vi "Begin.vi"   [LabVIEW 2011]
doc: "Called before other user functions, this VI is expected to open initial I/O refnums, load in file data, and do all program initialization. Notice that the <B>error out</B> terminal is simply used for data flow. Wiring it to other structures or subVIs ensures that this VI runs first."
uses:
  <vilib>/Rock Robotics/SystemInterfaces/DIO/FPGA_DIOPWMChannel.ctl
  <vilib>/Rock Robotics/SystemInterfaces/AI/FPGA_AIChannel.ctl
  <vilib>/Rock Robotics/WPI/Joystick/WPI_JoystickDeviceEnum.ctl
  Global.vi
  <vilib>/Rock Robotics/WPI/RobotDrive/WPI_RobotDriveOpen4MotorWithJaguar.vi
  Pivot Drive.lvlib
types:
  T1 = typedef "WPI_JoystickDeviceEnum.ctl" = enum16{"USB 1", "USB 2", "USB 3", "USB 4", "Kinect 1", "Kinect 2"}
  T2 = typedef "FPGA_AIChannel.ctl" = enum8{"AI 1", "AI 2", "AI 3", "AI 4", "AI 5", "AI 6", "AI 7", "AI 8", "Invalid"}
  T3 = typedef "FPGA_DIOPWMChannel.ctl" = enum8{"PWM 1", "PWM 2", "PWM 3", "PWM 4", "PWM 5", "PWM 6", "PWM 7", "PWM 8", "PWM 9", "PWM 10", "Invalid"}
  T4 = typedef "WPI_RobotDriveDevRef.ctl" = cluster{"DevStatus":errorcluster, "Motors[]":T5[], "Square Inputs":bool, "Max Output":dbl, "Isochronous":bool}
  T5 = typedef "WPI_MotorControlDeviceRef.ctl" = cluster{"DeviceStatus":errorcluster, "Type":enum16{"PWM", "CAN"}, "PWM":cluster{"Digital Module":T6, "PWM Channel":T3, "DeadBand":T7}, "CAN":cluster{"Device Number":u8, "Control Mode":T8, "Semaphore":T9, "Max Vout":dbl}, "Invert":bool, "TransformRef":T10, "InvTransformRef":T10}
  T6 = typedef "FPGA_TypedefDigitalModule.ctl" = enum16{"Digital Module 1", "Digital Module 2"}
  T7 = typedef "WPI_PWMDeadband.ctl" = cluster{"Name":string, "maxPositivePwm":i32, "minPositivePwm":i32, "centerPwm":i32, "maxNegativePwm":i32, "minNegativePwm":i32, "angularRange":u16}
  T8 = typedef "WPI_CANJaguar_ControlMode.ctl" = enum8{"Percent VBus", "Current", "Speed", "Position", "Voltage"}
  T9 = typedef "Semaphore RefNum" = refnum<k1>
  T10 = typedef "WPI_PWMTransform_ConPane.ctl" = refnum<vi>
  T11 = typedef "WPI_AnalogChannelDevRef.ctl" = cluster{"DevStatus":errorcluster, "Analog Module":T12, "Analog Channel":T2}
  T12 = typedef "FPGA_TypedefAnalogModule.ctl" = enum16{"Analog Module 1", "Analog Module 2"}
  T13 = typedef "WPI_JoystickDevRef.ctl" = cluster{"Device":T1}
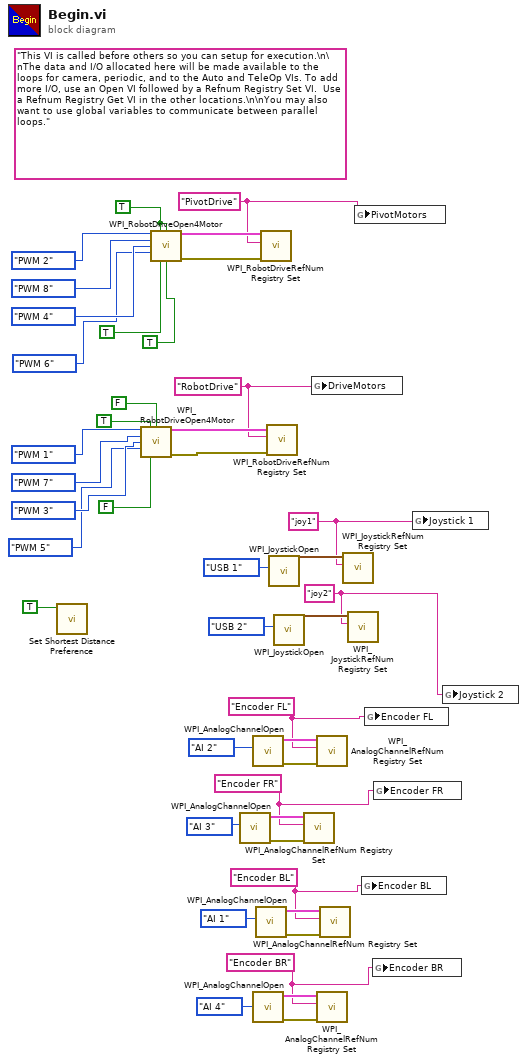
[diagram p0: block diagram]
diagram:
  w2 = TRUE ("Rear Left Motor Inverted")
  w24 = "joy2"
  w25 = "joy1"
  w16 = "Encoder BR" ("refnum name")
  w17 = "Encoder BL" ("refnum name")
  w18 = "Encoder FR" ("refnum name")
  w19 = "Encoder FL" ("refnum name")
  w20 = "RobotDrive" ("refnum name")
  w21 = "PivotDrive" ("refnum name")
  (unwired) "This VI is called before others so you can setup for execution.\n\nThe data and I/O allocated here will be made available to the loops for camera, periodic, and to the Auto and TeleOp VIs. To add more I/O, use an Open VI followed by a Refnum Registry Set VI.  Use a Refnum Registry Get VI in the other locations.\n\nYou may also want to use global variables to communicate between parallel loops."
  n1 = call "Set Shortest Distance Preference.vi"("Use Shortest Distance Relative?"=TRUE) -> ()  [unwired: 11 out]
  n2 = call-poly <vilib>:"WPI_RobotDriveOpen4Motor.vi"("Rear Left Motor"=FPGA_DIOPWMChannel."PWM 1", "Rear Left Motor Inverted"=TRUE ("Front Left Motor Inverted"), "Rear Right Motor Inverted"=FALSE, "Rear Right Motor"=FPGA_DIOPWMChannel."PWM 7" ("Rear Left Motor"), "Front Left Motor"=FPGA_DIOPWMChannel."PWM 3" ("Rear Left Motor"), "Front Right Motor"=FPGA_DIOPWMChannel."PWM 5" ("Rear Left Motor"), "Front Left Motor Inverted"=FALSE) -> ("RobotDriveDevRef"=w41:T4, "error out"=w40:errorcluster)  [unwired: 2 in, 5 out]
  n3 = call-poly <vilib>:"WPI_RobotDriveOpen4Motor.vi"("Rear Left Motor"=FPGA_DIOPWMChannel."PWM 2", "Rear Left Motor Inverted"=w2, "Rear Right Motor Inverted"=w2, "Rear Right Motor"=FPGA_DIOPWMChannel."PWM 8" ("Rear Left Motor"), "Front Left Motor"=FPGA_DIOPWMChannel."PWM 4" ("Rear Left Motor"), "Front Right Motor"=FPGA_DIOPWMChannel."PWM 6" ("Rear Left Motor"), "Front Left Motor Inverted"=TRUE, "Front Right Motor Inverted"=TRUE ("Front Left Motor Inverted")) -> ("RobotDriveDevRef"=w43:T4, "error out"=w42:errorcluster)  [unwired: 1 in, 5 out]
  n4 = call <vilib>:"WPI_AnalogChannelOpen.vi"("Analog Channel"=FPGA_AIChannel."AI 3") -> ("error out"=w37:errorcluster, "AIDeviceRef"=w36:T11)  [unwired: 2 in, 7 out]
  n5 = call <vilib>:"WPI_AnalogChannelOpen.vi"("Analog Channel"=FPGA_AIChannel."AI 2") -> ("error out"=w39:errorcluster, "AIDeviceRef"=w38:T11)  [unwired: 2 in, 7 out]
  n6 = call <vilib>:"WPI_AnalogChannelOpen.vi"("Analog Channel"=FPGA_AIChannel."AI 4") -> ("error out"=w33:errorcluster, "AIDeviceRef"=w32:T11)  [unwired: 2 in, 7 out]
  n7 = call <vilib>:"WPI_AnalogChannelOpen.vi"("Analog Channel"=FPGA_AIChannel."AI 1") -> ("error out"=w35:errorcluster, "AIDeviceRef"=w34:T11)  [unwired: 2 in, 7 out]
  n8 = call <vilib>:"WPI_RobotDriveRefNum Registry Set.vi"("error in (no error)"=w42, "refnum name"=w21, "RobotDriveDevRef"=w43) -> ()  [unwired: 9 out]
  n9 = call <vilib>:"WPI_RobotDriveRefNum Registry Set.vi"("error in (no error)"=w40, "refnum name"=w20, "RobotDriveDevRef"=w41) -> ()  [unwired: 9 out]
  n10 = call <vilib>:"WPI_JoystickOpen.vi"("JoystickDevice"=WPI_JoystickDeviceEnum."USB 1") -> ("JoystickDevRef"=w27:T13)  [unwired: 10 out]
  n11 = call <vilib>:"WPI_JoystickOpen.vi"("JoystickDevice"=WPI_JoystickDeviceEnum."USB 2") -> ("JoystickDevRef"=w26:T13)  [unwired: 10 out]
  n12 = call <vilib>:"WPI_AnalogChannelRefNum Registry Set.vi"("error in (no error)"=w37, "refnum name"=w18, "AIDeviceRef"=w36) -> ()  [unwired: 9 out]
  n13 = global write "Global.vi" "DriveMotors"(w20) -> ()
  n14 = call <vilib>:"WPI_AnalogChannelRefNum Registry Set.vi"("error in (no error)"=w39, "refnum name"=w19, "AIDeviceRef"=w38) -> ()  [unwired: 9 out]
  n15 = call <vilib>:"WPI_AnalogChannelRefNum Registry Set.vi"("error in (no error)"=w33, "refnum name"=w16, "AIDeviceRef"=w32) -> ()  [unwired: 9 out]
  n16 = call <vilib>:"WPI_AnalogChannelRefNum Registry Set.vi"("error in (no error)"=w35, "refnum name"=w17, "AIDeviceRef"=w34) -> ()  [unwired: 9 out]
  n17 = call <vilib>:"WPI_JoystickRefNum Registry Set.vi"("refnum name"=w25, "JoystickDevRef"=w27) -> ()  [unwired: 1 in, 9 out]
  n18 = call <vilib>:"WPI_JoystickRefNum Registry Set.vi"("refnum name"=w24, "JoystickDevRef"=w26) -> ()  [unwired: 1 in, 9 out]
  n19 = global write "Global.vi" "PivotMotors"(w21) -> ()
  n20 = global write "Global.vi" "Encoder BL"(w17) -> ()
  n21 = global write "Global.vi" "Encoder FL"(w19) -> ()
  n22 = global write "Global.vi" "Encoder BR"(w16) -> ()
  n23 = global write "Global.vi" "Encoder FR"(w18) -> ()
  n24 = global write "Global.vi" "Joystick 1"(w25) -> ()
  n25 = global write "Global.vi" "Joystick 2"(w24) -> ()
